vi "Field_Step.vi"   [LabVIEW 2016]
uses:
  Global/Global Variables/global.vi
  Global/Global Variables/Data_Display_global.vi
  Instrument_Setup.vi
types:
  T1 = typedef "PSIO.ctl" = cluster{"Address":T2, "Version":enum16{"PS", "IPS"}}
  T2 = typedef "OxfordAddress.ctl" = cluster{"Com Port":i32, "ISOBUS Address":i32, "GPIB Address":i16, "Communication":enum16{"RS232", "ISOBUS", "GPIB", "Gateway"}}
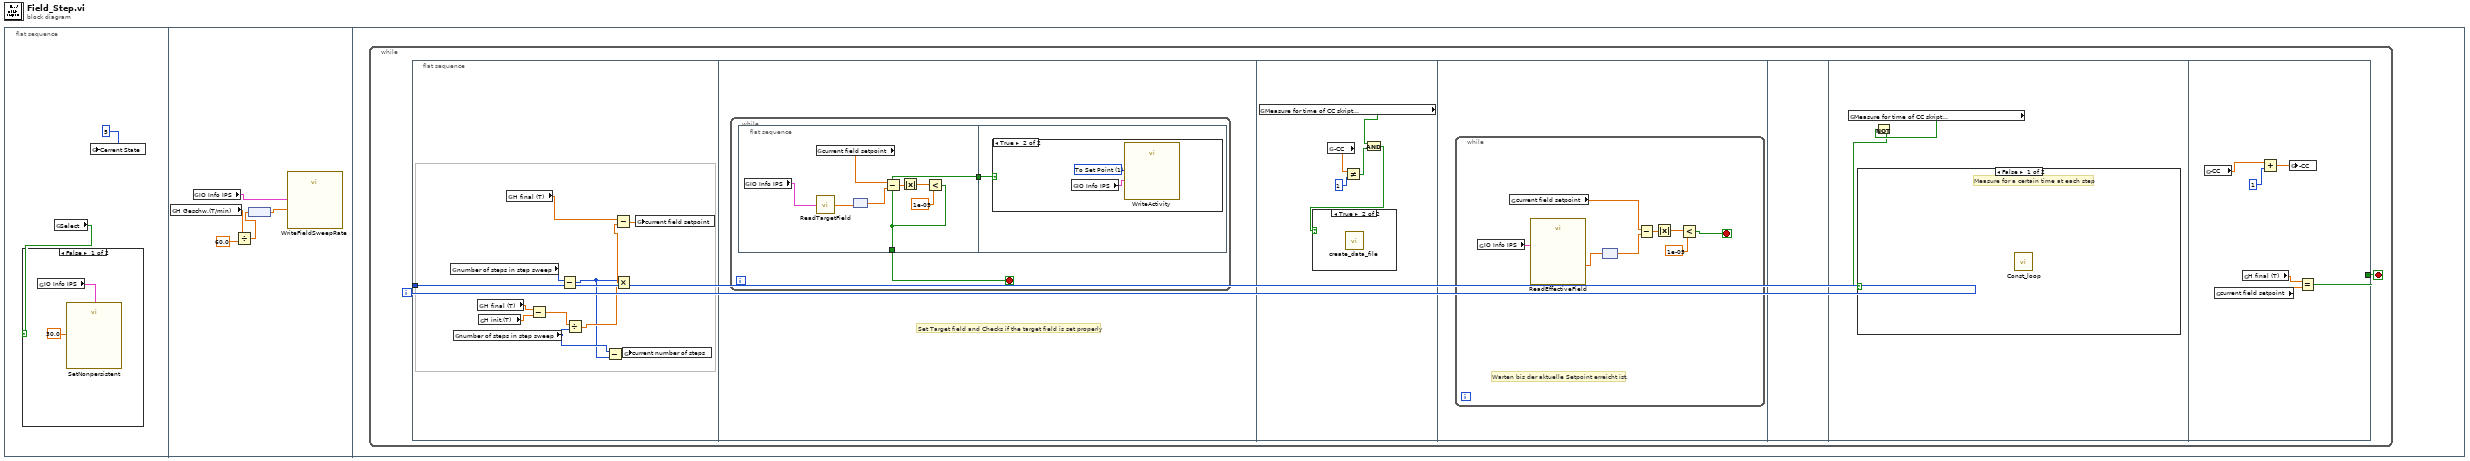
[diagram p0: block diagram]
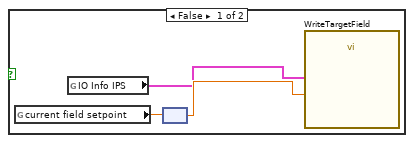
[diagram p3: hidden frame]
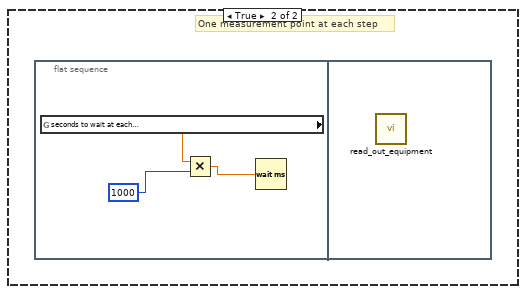
[diagram p5: hidden frame]
diagram:
  n1 = flat-sequence {
    frame #0 {
      n2 = global read "Data_Display_global.vi" "Select"() -> (w1:bool)
      n3 = case shown="False" w1 {
        frame False {
          n4 = global read "Instrument_Setup.vi" "IO Info IPS"() -> (w4:T1)
          n5 = call "SetNonpersistent.vi"("Switch Heater Dwell Time"=dbl[unit] 30.0, "IO Info"=w4) -> ()  [unwired: 2 out]
        }
        frame True {
        }
      }
      n6 = global write "global.vi" "Cerrent State"(5) -> ()
    }
    frame #1 {
      n7 = global read "global.vi" "H Geschw.(T/min)"() -> (w7:dbl)
      n8 = global read "Instrument_Setup.vi" "IO Info IPS"() -> (w9:T1)
      n9 = Divide(x=w7, y=60.0) -> (x/y=w5:dbl)
      n10 = node(w5) -> (w8:dbl[unit])
      n11 = call "WriteFieldSweepRate.vi"("Sweep rate"=w8, "IO Info"=w9) -> ()  [unwired: 1 out]
    }
    frame #2 {
      n12 = while {
        i -> [w11]
        stop <- w10 stop-if-true
        n13 = flat-sequence {
          tunnel: w11 -> [w20]
          tunnel: [w62] -> w10
          frame #0 {
            n14 = global read "global.vi" "number of steps in step sweep"() -> (w18:i32)
            n15 = global read "global.vi" "number of steps in step sweep"() -> (w16:i32)
            n16 = global read "global.vi" "H final (T)"() -> (w14:dbl)
            n17 = global read "global.vi" "H init.(T)"() -> (w13:dbl)
            n18 = global read "global.vi" "H final (T)"() -> (w23:dbl)
            n19 = Subtract(x=w14, y=w13) -> (x-y=w12:dbl)
            n20 = Subtract(x=w18, y=w20) -> (x-y=w15:i32)
            n21 = Divide(x=w12, y=w16) -> (x/y=w21:dbl)
            n22 = Subtract(x=w16, y=w15) -> (x-y=w17:i32)
            n23 = Multiply(x=w15, y=w21) -> (x*y=w22:dbl)
            n24 = Subtract(x=w23, y=w22) -> (x-y=w19:dbl)
            n25 = global write "Data_Display_global.vi" "current number of steps"(w17) -> ()
            n26 = global write "Data_Display_global.vi" "current field setpoint"(w19) -> ()
          }
          frame #1 {
            # "Set Target field and Checks if the target field is set properly"
            n27 = while {
              stop <- w24 stop-if-true
              n28 = flat-sequence {
                tunnel: [w26] -> w25
                tunnel: [w26] -> w24
                tunnel: w25 -> [w34]
                frame #0 {
                  n29 = global read "Instrument_Setup.vi" "IO Info IPS"() -> (w33:T1)
                  n30 = global read "Data_Display_global.vi" "current field setpoint"() -> (w27:dbl)
                  n31 = call "ReadTargetField.vi"("IO Info"=w33) -> ("Target field"=w32:dbl[unit])  [unwired: 2 out]
                  n32 = node(w32) -> (w28:dbl)
                  n33 = Subtract(x=w27, y=w28) -> (x-y=w30:dbl)
                  n34 = Absolute Value(x=w30) -> (abs(x)=w29:dbl)
                  n35 = Less?(x=w29, y=1e-05) -> (x < y?=w26:bool)
                }
                frame #1 {
                  n36 = case shown="True" w34 {
                    frame False {
                      n37 = global read "Data_Display_global.vi" "current field setpoint"() -> (w37:dbl)
                      n38 = global read "Instrument_Setup.vi" "IO Info IPS"() -> (w35:T1)
                      n39 = node(w37) -> (w36:dbl[unit])
                      n40 = call "WriteTargetField.vi"("Target Field"=w36, "IO Info"=w35) -> ()  [unwired: 1 in, 1 out]
                    }
                    frame True {
                      w39 = u16 1 items=["Hold", "To Set Point", "To Zero", "Clamp"] ("Activity")
                      n41 = global read "Instrument_Setup.vi" "IO Info IPS"() -> (w38:T1)
                      n42 = call "WriteActivity.vi"("Activity"=w39, "IO Info"=w38) -> ()  [unwired: 1 in, 1 out]
                    }
                  }
                }
              }
            }
          }
          frame #2 {
            n43 = global read "Instrument_Setup.vi" "Measure for time of CC skript\nat each field step point"() -> (w42:bool)
            n44 = global read "global.vi" "-CC"() -> (w44:dbl)
            n45 = Not Equal?(x=w44, y=1) -> (x != y?=w41:bool)
            n46 = And(x=w42, y=w41) -> (x .and. y?=w40:bool)
            n47 = case shown="True" w40 {
              frame False {
              }
              frame True {
                n48 = call "create_data_file.vi"() -> ()  [unwired: 3 in]
              }
            }
          }
          frame #3 {
            n49 = while {
              stop <- w47 stop-if-true
              # "Warten bis der aktuelle Setpoint erreicht ist."
              n50 = global read "Instrument_Setup.vi" "IO Info IPS"() -> (w52:T1)
              n51 = global read "Data_Display_global.vi" "current field setpoint"() -> (w50:dbl)
              n52 = call "ReadEffectiveField.vi"("IO Info"=w52) -> ("Effective field"=w51:dbl[unit])  [unwired: 2 out]
              n53 = node(w51) -> (w49:dbl)
              n54 = Subtract(x=w50, y=w49) -> (x-y=w46:dbl)
              n55 = Absolute Value(x=w46) -> (abs(x)=w45:dbl)
              n56 = Less?(x=w45, y=1e-05) -> (x < y?=w47:bool)
            }
          }
          frame #4 {
          }
          frame #5 {
            n57 = global read "Instrument_Setup.vi" "Measure for time of CC skript\nat each field step point"() -> (w54:bool)
            n58 = Not(x=w54) -> (.not. x?=w53:bool)
            n59 = case shown="False" w53 {
              frame False {
                # "Measure for a certain time at each step"
                n60 = call "Const_loop.vi"() -> ()  [unwired: 4 in]
              }
              frame True {
                # "One measurement point at each step"
                n61 = flat-sequence {
                  frame #0 {
                    n62 = global read "Instrument_Setup.vi" "seconds to wait at each\nfield step in a step sweep"() -> (w57:dbl)
                    n63 = Multiply(x=w57, y=u32 1000 ("milliseconds to wait")) -> (x*y=w55:dbl)
                    n64 = Wait (ms)(milliseconds to wait=w55) -> ()  [unwired: 1 out]
                  }
                  frame #1 {
                    n65 = call "read_out_equipment.vi"() -> ()  [unwired: 1 in]
                  }
                }
              }
            }
          }
          frame #6 {
            n66 = global read "global.vi" "-CC"() -> (w60:dbl)
            n67 = global read "Data_Display_global.vi" "current field setpoint"() -> (w61:dbl)
            n68 = global read "global.vi" "H final (T)"() -> (w63:dbl)
            n69 = Add(x=w60, y=1) -> (x+y=w58:dbl)
            n70 = global write "global.vi" "-CC"(w58) -> ()
            n71 = Equal?(x=w63, y=w61) -> (x = y?=w62:bool)
          }
        }
      }
    }
  }
